vi "PrepareData.vi"(8 "Filtering settings":T1, 9 "Calibration factors":cluster{"x":dbl, "y":dbl, "z":dbl}, 10 "Sampling frequecy":dbl, 11 "3 axis + tacho":waveform(dbl)[](array[waveform])) -> (3 "3 axis + frequency":T2)   [LabVIEW 2019]
uses:
  <vilib>/Analysis/3filter.llb/Filter Passband Type.ctl
  <vilib>/measure/madcrms.llb/Basic Averaged DC-RMS for 1 Chan.vi
  <vilib>/measure/mascope.llb/Pulse Measurements 1 chan.vi
  <vilib>/Analysis/3filter.llb/Butterworth Filter (DBL).vi
  <vilib>/measure/NI_MAPro.lvlib
  <vilib>/Analysis/NI_AALBase.lvlib
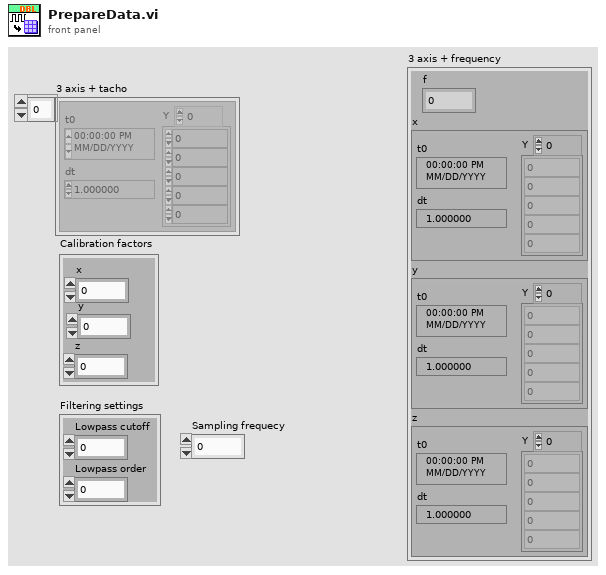
[diagram p1: front panel]
types:
  T1 = cluster{"Lowpass cutoff":dbl, "Lowpass order":i32}
  T2 = cluster{"f":dbl, "x":waveform(dbl), "y":waveform(dbl), "z":waveform(dbl)}
  T3 = typedef "NI_AALBase.lvlib/Filter Passband Type.ctl" = enum32{"Lowpass", "Highpass", "Bandpass", "Bandstop"}
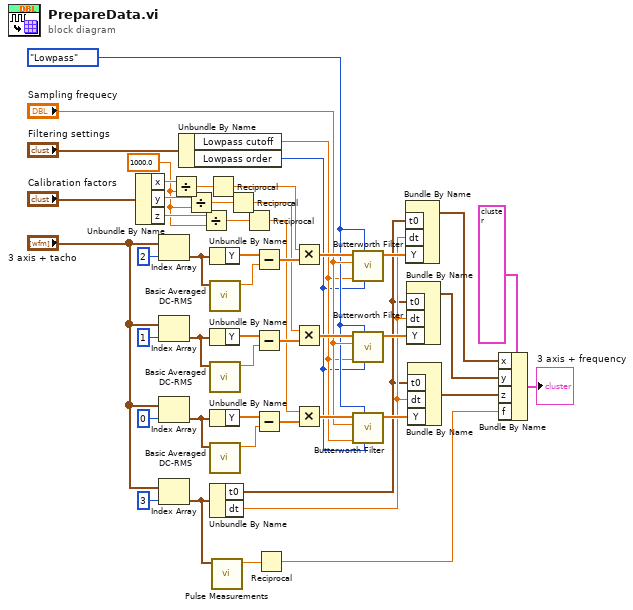
[diagram p0: block diagram]
diagram:
  w4 = 1000.0 ("y")
  w24 = Filter_Passband_Type."Lowpass" ("filter type")
  n1 = Unbundle By Name("Calibration factors") -> ("x"=w10:dbl, "y"=w5:dbl, "z"=w9:dbl)
  n2 = Index Array(array="3 axis + tacho", index=2) -> (element=w39:waveform(dbl))
  n3 = Index Array(array="3 axis + tacho", index=1) -> (element=w40:waveform(dbl))
  n4 = Index Array(array="3 axis + tacho", index=0) -> (element=w41:waveform(dbl))
  n5 = Index Array(array="3 axis + tacho", index=3) -> (element=w37:waveform(dbl))
  n6 = Divide(x=w10, y=w4) -> (x/y=w8:dbl)
  n7 = Unbundle By Name("Filtering settings") -> ("Lowpass cutoff"=w13:dbl, "Lowpass order"=w12:i32)
  n8 = Divide(x=w5, y=w4) -> (x/y=w7:dbl)
  n9 = Divide(x=w9, y=w4) -> (x/y=w6:dbl)
  n10 = Reciprocal(x=w8) -> (1/x=w3:dbl)
  n11 = Unbundle By Name(w39) -> ("Y"=w34:dbl[])
  n12 = call-poly <vilib>:"Basic Averaged DC-RMS.vi"("signal in"=w39) -> ("DC value"=w49:dbl)  [unwired: 7 in, 3 out]
  n13 = Unbundle By Name(w40) -> ("Y"=w33:dbl[])
  n14 = call-poly <vilib>:"Basic Averaged DC-RMS.vi"("signal in"=w40) -> ("DC value"=w48:dbl)  [unwired: 7 in, 3 out]
  n15 = Unbundle By Name(w41) -> ("Y"=w32:dbl[])
  n16 = call-poly <vilib>:"Basic Averaged DC-RMS.vi"("signal in"=w41) -> ("DC value"=w47:dbl)  [unwired: 7 in, 3 out]
  n17 = Unbundle By Name(w37) -> ("t0"=w19:timestamp, "dt"=w20:dbl)
  n18 = call-poly <vilib>:"Pulse Measurements.vi"("signal in"=w37) -> ("period"=w36:dbl)  [unwired: 6 in, 4 out]
  n19 = Reciprocal(x=w7) -> (1/x=w2:dbl)
  n20 = Reciprocal(x=w6) -> (1/x=w1:dbl)
  n21 = Subtract(x=w34, y=w49) -> (x-y=w31:dbl[])
  n22 = Subtract(x=w33, y=w48) -> (x-y=w30:dbl[])
  n23 = Subtract(x=w32, y=w47) -> (x-y=w29:dbl[])
  n24 = Reciprocal(x=w36) -> (1/x=w35:dbl)
  n25 = Multiply(x=w3, y=w31) -> (x*y=w28:dbl[])
  n26 = Multiply(x=w2, y=w30) -> (x*y=w27:dbl[])
  n27 = Multiply(x=w1, y=w29) -> (x*y=w26:dbl[])
  n28 = call-poly <vilib>:"Butterworth Filter.vi"("order"=w12, "filter type"=w24, "low cutoff freq: fl"=w13, "sampling freq: fs"="Sampling frequecy", "X"=w28) -> ("Filtered X"=w23:dbl[])  [unwired: 3 in, 1 out]
  n29 = call-poly <vilib>:"Butterworth Filter.vi"("order"=w12, "filter type"=w24, "low cutoff freq: fl"=w13, "sampling freq: fs"="Sampling frequecy", "X"=w27) -> ("Filtered X"=w22:dbl[])  [unwired: 3 in, 1 out]
  n30 = call-poly <vilib>:"Butterworth Filter.vi"("order"=w12, "filter type"=w24, "low cutoff freq: fl"=w13, "sampling freq: fs"="Sampling frequecy", "X"=w26) -> ("Filtered X"=w21:dbl[])  [unwired: 3 in, 1 out]
  n31 = Bundle By Name("t0"=w19, "dt"=w20, "Y"=w23) -> (w16:waveform(dbl))  [unwired: 1 in]
  n32 = Bundle By Name("t0"=w19, "dt"=w20, "Y"=w22) -> (w17:waveform(dbl))  [unwired: 1 in]
  n33 = Bundle By Name("t0"=w19, "dt"=w20, "Y"=w21) -> (w18:waveform(dbl))  [unwired: 1 in]
  n34 = Bundle By Name(cluster=T2 {"f"=0.0, "x"={"t0"=timestamp(0 s since 1904-01-01), "dt"=1.0, "Y"=[]}, "y"={"t0"=timestamp(0 s since 1904-01-01), "dt"=1.0, "Y"=[]}, "z"={"t0"=timestamp(0 s since 1904-01-01), "dt"=1.0, "Y"=[]}} ("input cluster"), "x"=w16, "y"=w17, "z"=w18, "f"=w35) -> (→"3 axis + frequency":T2)
